vi "note_array.to_pictures.vi"() -> ()   [LabVIEW 2020, in "midi-ui.lvclass"]
uses:
  midi-ui.lvclass
  midi-ui.lvclass/midi-ui.ctl
panel:
  in  "Note Off Colour":u32(colorbox)=6618880
  in  "Note Array":T1(array[cluster])
  out "midi-ui out":refnum<class "midi-ui.lvclass">
  in  "midi-ui in":refnum<class "midi-ui.lvclass">
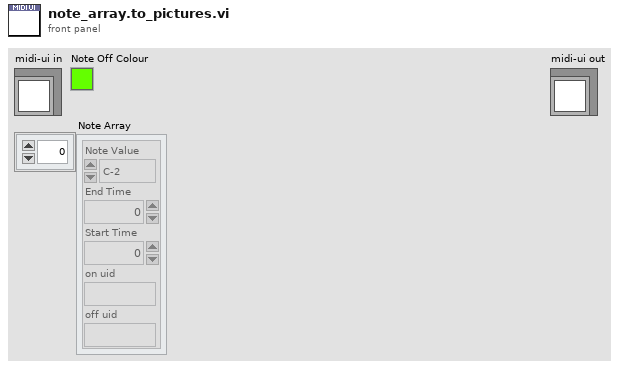
[diagram p1: front panel]
types:
  T1 = cluster{"Note Value":enum8{"C-2", "C#-2", "D-2", "D#-2", "E-2", "F-2", "F#-2", "G-2", "G#-2", "A-2", "A#-2", "B-2", "C-1", "C#-1", "D-1", "D#-1", "E-1", "F-1", "F#-1", "G-1", "G#-1", "A-1", "A#-1", "B-1", "C0", "C#0", "D0", "D#0", "E0", "F0", "F#0", "G0", "G#0", "A0", "A#0", "B0", "C1", "C#1", "D1", "D#1", "E1", "F1", "F#1", "G1", "G#1", "A1", "A#1", "B1", "C2", "C#2", "D2", "D#2", "E2", "F2", "F#2", "G2", "G#2", "A2", "A#2", "B2", "C3", "C#3", "D3", "D#3", "E3", "F3", "F#3", "G3", "G#3", "A3", "A#3", "B3", "C4", "C#4", "D4", "D#4", "E4", "F4", "F#4", "G4", "G#4", "A4", "A#4", "B4", "C5", "C#5", "D5", "D#5", "E5", "F5", "F#5", "G5", "G#5", "A5", "A#5", "B5", "C6", "C#6", "D6", "D#6", "E6", "F6", "F#6", "G6", "G#6", "A6", "A#6", "B6", "C7", "C#7", "D7", "D#7", "E7", "F7", "F#7", "G7", "G#7", "A7", "A#7", "B7", "C8", "C#8", "D8", "D#8", "E8", "F8", "F#8", "G"}, "End Time":u32, "Start Time":u32, "on uid":string, "off uid":string}[]
  T2 = map{i32, cluster{"Note On":picture, "Note Off":picture}}
  T3 = cluster{"left":i16, "top":i16, "right":i16, "bottom":i16}
  T4 = enum8{"C-2", "C#-2", "D-2", "D#-2", "E-2", "F-2", "F#-2", "G-2", "G#-2", "A-2", "A#-2", "B-2", "C-1", "C#-1", "D-1", "D#-1", "E-1", "F-1", "F#-1", "G-1", "G#-1", "A-1", "A#-1", "B-1", "C0", "C#0", "D0", "D#0", "E0", "F0", "F#0", "G0", "G#0", "A0", "A#0", "B0", "C1", "C#1", "D1", "D#1", "E1", "F1", "F#1", "G1", "G#1", "A1", "A#1", "B1", "C2", "C#2", "D2", "D#2", "E2", "F2", "F#2", "G2", "G#2", "A2", "A#2", "B2", "C3", "C#3", "D3", "D#3", "E3", "F3", "F#3", "G3", "G#3", "A3", "A#3", "B3", "C4", "C#4", "D4", "D#4", "E4", "F4", "F#4", "G4", "G#4", "A4", "A#4", "B4", "C5", "C#5", "D5", "D#5", "E5", "F5", "F#5", "G5", "G#5", "A5", "A#5", "B5", "C6", "C#6", "D6", "D#6", "E6", "F6", "F#6", "G6", "G#6", "A6", "A#6", "B6", "C7", "C#7", "D7", "D#7", "E7", "F7", "F#7", "G7", "G#7", "A7", "A#7", "B7", "C8", "C#8", "D8", "D#8", "E8", "F8", "F#8", "G"}
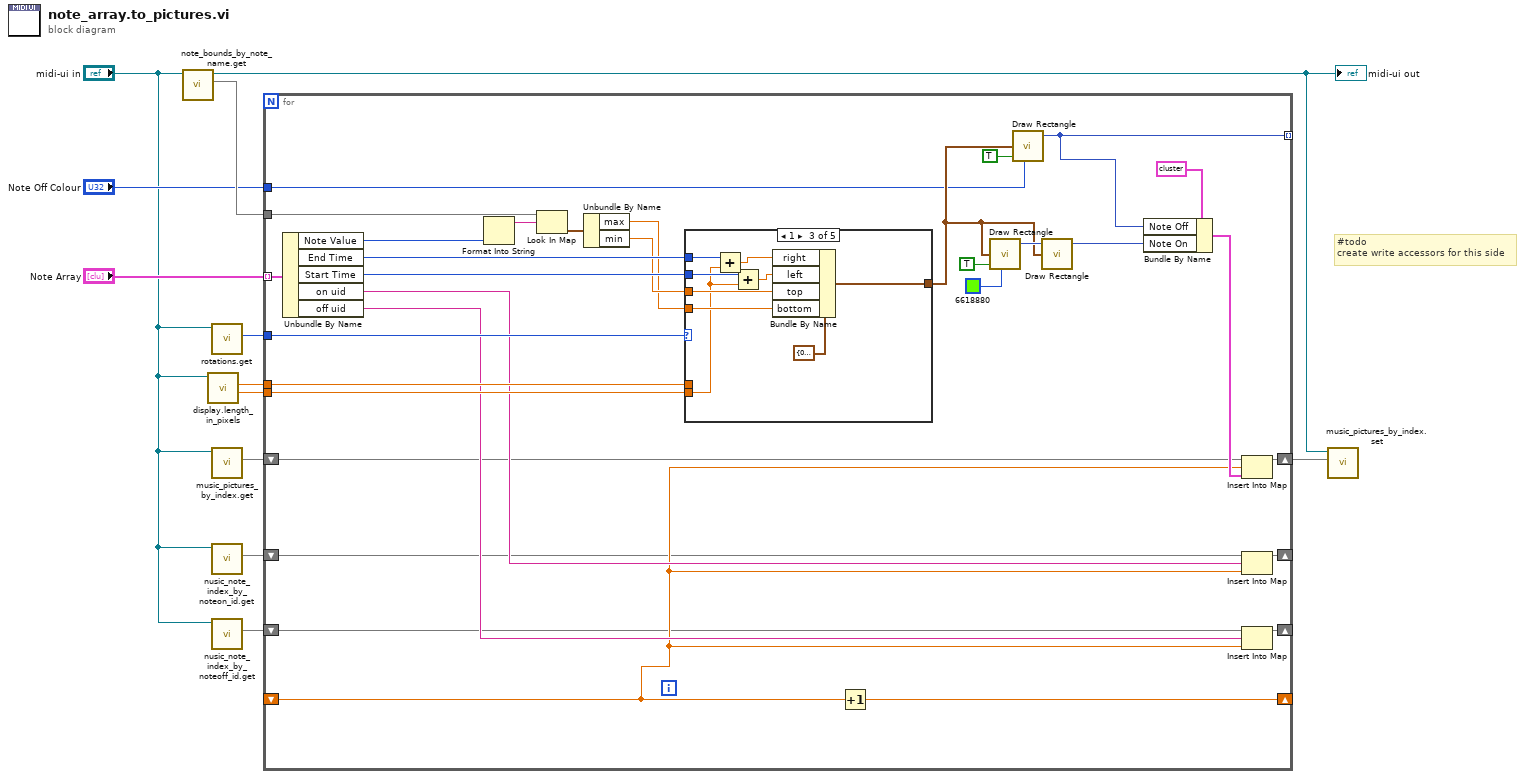
[diagram p0: block diagram]
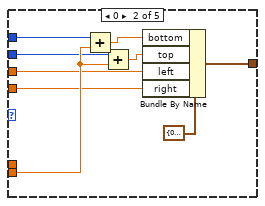
[diagram p3: hidden frame]
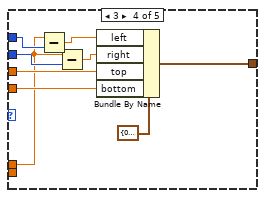
[diagram p4: hidden frame]
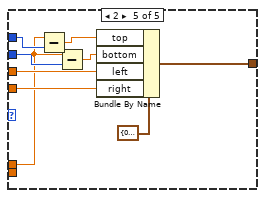
[diagram p5: hidden frame]
diagram:
  # "#todo\ncreate write accessors for this side"
  n1 = call "note_bounds_by_note_name.get.vi"("midi-ui in"="midi-ui in") -> ("Note Bounds by Note Name"=w12:map{string, cluster{"max":dbl, "min":dbl}}, "midi-ui out"=w1:refnum<class "midi-ui.lvclass">)  [unwired: 8 in, 1 out]
  "midi-ui out" <- w1
  n2 = call "display.length_in_pixels.vi"("midi-ui in"="midi-ui in") -> ("White Key Length (px)"=w5:dbl, "note board Length (px)"=w4:dbl)  [unwired: 7 in, 2 out]
  n3 = call "rotations.get.vi"("midi-ui in"="midi-ui in") -> ("Anticlockwise rotations [0-3] (0)"=w10:i32)  [unwired: 8 in, 2 out]
  n4 = call "music_pictures_by_index.get.vi"("midi-ui in"="midi-ui in") -> ("Music Pictures by Index"=w9:T2)  [unwired: 8 in, 2 out]
  n5 = call "nusic_note_index_by_noteon_id.get.vi"("midi-ui in"="midi-ui in") -> ("Music Note Index by NoteOnID"=w6:map{string, i32})  [unwired: 8 in, 2 out]
  n6 = call "nusic_note_index_by_noteoff_id.get.vi"("midi-ui in"="midi-ui in") -> ("Music Note Index by NoteOffID"=w7:map{string, i32})  [unwired: 8 in, 2 out]
  n7 = for {
    tunnel: "Note Array" -> [w44] mode=indexing
    tunnel: w12 -> [w22]
    tunnel: w10 -> [w37]
    tunnel: w5 -> [w36]
    tunnel: w4 -> [w35]
    shift-right: [w33] -> _
    shift-left: w6 -> [w17]
    shift-right: [w24] -> _
    shift-left: w7 -> [w16]
    tunnel: [w20] -> _ mode=indexing
    shift-right: [w19] -> _
    shift-left: _ -> [w18]
    shift-right: [w14] -> w2
    shift-left: w9 -> [w15]
    tunnel: "Note Off Colour" -> [w13]
    n8 = Unbundle By Name(w44) -> ("Note Value"=w40:T4, "End Time"=w42:u32, "Start Time"=w43:u32, "on uid"=w25:string, "off uid"=w23:string)
    n9 = Format Into String(w40) -> (resulting string=w34:string)  [unwired: 3 in, 1 out]
    n10 = Look In Map(map=w22, key=w34) -> (value=w41:cluster{"max":dbl, "min":dbl})  [unwired: 1 in, 1 out]
    n11 = Unbundle By Name(w41) -> ("max"=w38:dbl, "min"=w39:dbl)
    n12 = case shown="1" w37 {
      tunnel: w43 -> [_ w48 w57 w66 w75]
      tunnel: w42 -> [_ w50 w58 w67 w76]
      tunnel: [_ w45 w61 w70 w79] -> w28
      tunnel: w39 -> [_ w47 w60 w69 w78]
      tunnel: w38 -> [_ w46 w59 w68 w77]
      tunnel: w36 -> [_ w49 w54 _ _]
      tunnel: w35 -> [_ _ _ w63 w72]
      frame Default {
      }
      frame 0 {
        n13 = Add(x=w50, y=w49) -> (x+y=w52:dbl)
        n14 = Add(x=w48, y=w49) -> (x+y=w51:dbl)
        n15 = Bundle By Name(cluster=T3 {"left"=0, "top"=0, "right"=0, "bottom"=0} ("rect"), "bottom"=w52, "top"=w51, "left"=w47, "right"=w46) -> (w45:T3)
      }
      frame 1 {
        n16 = Add(x=w58, y=w54) -> (x+y=w56:dbl)
        n17 = Add(x=w57, y=w54) -> (x+y=w55:dbl)
        n18 = Bundle By Name(cluster=T3 {"left"=0, "top"=0, "right"=0, "bottom"=0} ("rect"), "right"=w56, "left"=w55, "top"=w60, "bottom"=w59) -> (w61:T3)
      }
      frame 3 {
        n19 = Subtract(x=w63, y=w67) -> (x-y=w65:dbl)
        n20 = Subtract(x=w63, y=w66) -> (x-y=w64:dbl)
        n21 = Bundle By Name(cluster=T3 {"left"=0, "top"=0, "right"=0, "bottom"=0} ("rect"), "left"=w65, "right"=w64, "top"=w69, "bottom"=w68) -> (w70:T3)
      }
      frame 2 {
        n22 = Subtract(x=w72, y=w76) -> (x-y=w74:dbl)
        n23 = Subtract(x=w72, y=w75) -> (x-y=w73:dbl)
        n24 = Bundle By Name(cluster=T3 {"left"=0, "top"=0, "right"=0, "bottom"=0} ("rect"), "top"=w74, "bottom"=w73, "left"=w78, "right"=w77) -> (w79:T3)
      }
    }
    n25 = Increment(x=w18) -> (x+1=w19:dbl)
    n26 = call <vilib>:"Draw Rectangle.vi"("rect"=w28, "fill?(F)"=TRUE, "color(black)"=u32 6618880) -> ("new picture"=w29:picture)  [unwired: 6 in]
    n27 = call <vilib>:"Draw Rectangle.vi"("rect"=w28, "fill?(F)"=TRUE, "color(black)"=w13) -> ("new picture"=w20:picture)  [unwired: 6 in]
    n28 = call <vilib>:"Draw Rectangle.vi"("picture"=w29, "rect"=w28) -> ("new picture"=w27:picture)  [unwired: 7 in]
    n29 = Bundle By Name(cluster=cluster{"Note On":picture, "Note Off":picture} {"Note On"=bytes[0], "Note Off"=bytes[0]} ("value"), "Note Off"=w20, "Note On"=w27) -> (w26:cluster{"Note On":picture, "Note Off":picture})
    n30 = Insert Into Map(map in=w15, key=w18, value=w26) -> (map out=w14:T2)  [unwired: 2 out]
    n31 = Insert Into Map(map in=w17, key=w25, value=w18) -> (map out=w33:map{string, i32})  [unwired: 2 out]
    n32 = Insert Into Map(map in=w16, key=w23, value=w18) -> (map out=w24:map{string, i32})  [unwired: 2 out]
  }
  n33 = call "music_pictures_by_index.set.vi"("Music Pictures by Index"=w2, "midi-ui in"=w1) -> ()  [unwired: 8 in, 2 out]
